vi "PNG.vi"(7 "Current PNG filename":string, 8 "error in (no error)":errorcluster, 11 "Folder path":path) -> (0 "error out":errorcluster, 1 "Height":i16, 2 "Width":i16, 3 "2D Pixmap":u32[][](array[numeric]) format="%x", 4 "PNG Picture":picture, 6 "Cluster":cluster{"Width":dbl, "Height":dbl})   [LabVIEW 2023]
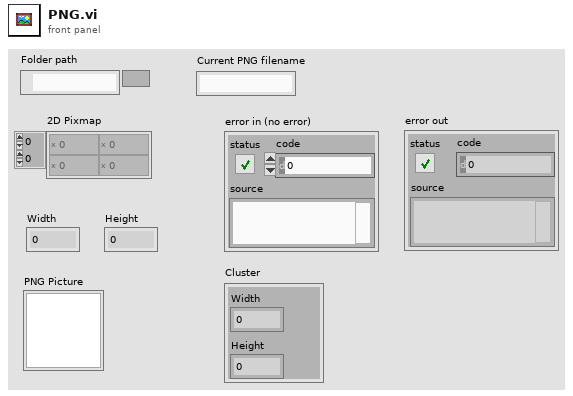
[diagram p1: front panel]
types:
  T1 = typedef "imagedata.ctl" = cluster{"image type":i32, "image depth":i32, "image":u8[], "mask":u8[], "colors":u32[], "Rectangle":cluster{"left":i16, "top":i16, "right":i16, "bottom":i16}}
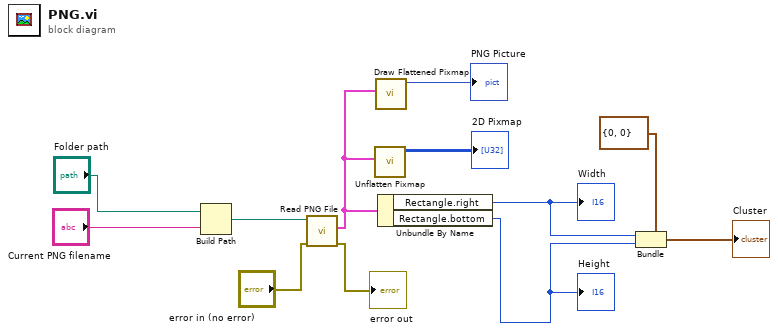
[diagram p0: block diagram]
diagram:
  n1 = Build Path(base path="Folder path", name or relative path="Current PNG filename") -> (appended path=w10:path)
  n2 = call <vilib>:"Read PNG File.vi"("error in (no error)"="error in (no error)", "path to PNG file"=w10) -> ("error out"=→"error out":errorcluster, "image data"=w7:T1)  [unwired: 7 in, 1 out]
  n3 = call <vilib>:"Unflatten Pixmap.vi"("image data"=w7) -> ("24-bit pixmap"=→"2D Pixmap":u32[][])  [unwired: 4 in, 6 out]
  n4 = call <vilib>:"Draw Flattened Pixmap.vi"("image data"=w7) -> ("new picture"=→"PNG Picture":picture)  [unwired: 8 in]
  n5 = Unbundle By Name(w7) -> ("Rectangle.right"=w6:i16, "Rectangle.bottom"=w2:i16)
  "Width" <- w6
  "Height" <- w2
  n6 = Bundle(cluster=cluster{i32, i32} {0, 0}, w6, w2) -> (→"Cluster":cluster{i32, i32})
